vi "Tab Test.vi"(11 "Name":string) -> ()   [LabVIEW 2018, in "Tab.lvlib"]
uses:
  Tab.lvlib
panel:
  out "current time":timestamp
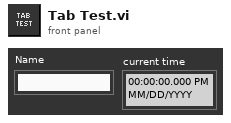
[diagram p1: front panel]
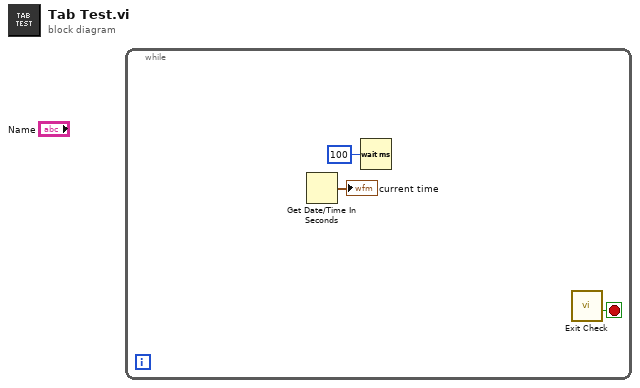
[diagram p0: block diagram]
diagram:
  n1 = while {
    stop <- w3 stop-if-true
    n2 = Get Date/Time In Seconds() -> (seconds since 1Jan1904=→"current time":timestamp)
    n3 = Wait (ms)(milliseconds to wait=u32 100) -> ()  [unwired: 1 out]
    n4 = call "Exit Check.vi"() -> ("Exit?"=w3:bool)  [unwired: 10 in, 1 out]
  }
